vi "zad71.vi"() -> ()   [LabVIEW 2018]
uses:
  ProductsCluster.ctl
  ProductsDataToWork.ctl
  ProgramStates.ctl
  <vilib>/Utility/file.llb/Read Delimited Spreadsheet (string).vi
panel:
  in  "?":bool
  in  "SortBy":enum16{"Name", "Number", "Producer"}(ring)
  in  "?":bool
  in  "?":bool
  in  "?":bool
  in  "?":bool
  in  "Search Value":string
  in  "SearchBy":enum16{"Name", "Number", "Producer"}(ring)=enum."Number"
  in  "?":bool
  in  "?":bool
  in  "?":bool
  in  "?":bool
  out "?":T1={"Numer Produktu"="1112", "Nazwa Produktu"="Laptop", "Wytwórca"="Dell"}
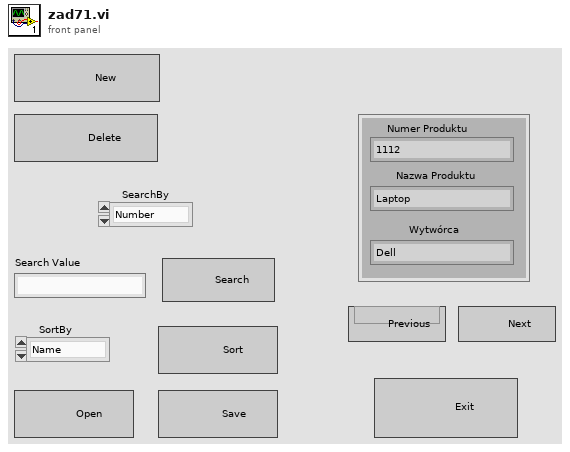
[diagram p1: front panel]
types:
  T1 = typedef "ProductsCluster.ctl" = cluster{"Numer Produktu":string, "Nazwa Produktu":string, "Wytwórca":string}
  T2 = typedef "ProductsDataToWork.ctl" = cluster{"Products":T1[], "CurrentProduct":i32, "SearchBy":enum16{"Name", "Number", "Producer"}, "SearchValue":string, "DataFilePath":path, "SortBy":enum16{"Name", "Number", "Producer"}}
  T3 = typedef "ProgramStates.ctl" = enum16{"Init", "Idle", "Open", "ShowPrevorious", "ShowNext", "Search", "Sort", "Add", "Delete", "Save", "Exit"}
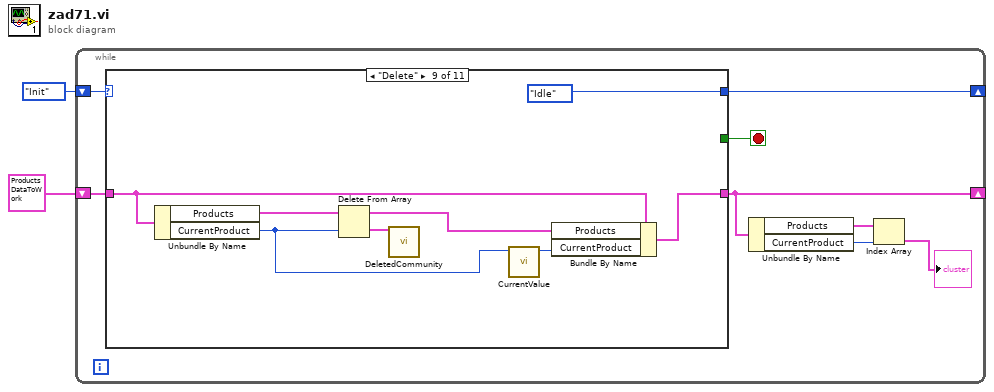
[diagram p0: block diagram]
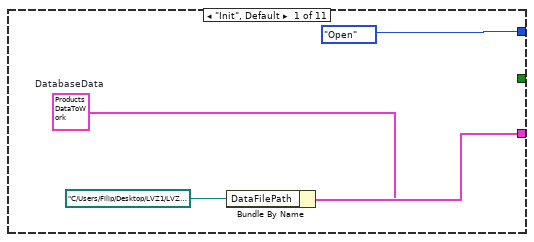
[diagram p2: hidden frame]
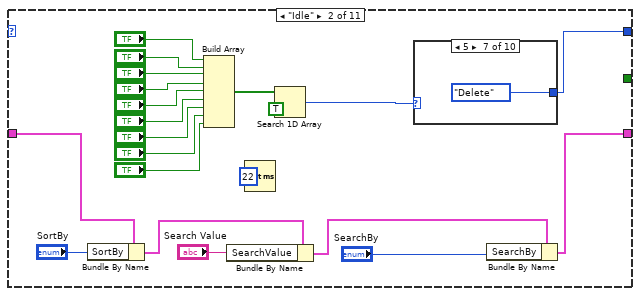
[diagram p3: hidden frame]
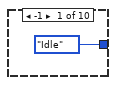
[diagram p4: hidden frame]
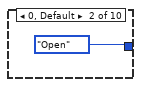
[diagram p5: hidden frame]
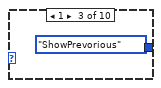
[diagram p6: hidden frame]
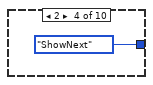
[diagram p7: hidden frame]
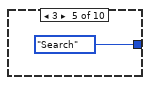
[diagram p8: hidden frame]
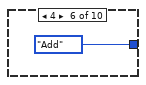
[diagram p9: hidden frame]
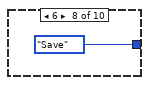
[diagram p10: hidden frame]
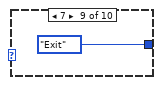
[diagram p11: hidden frame]
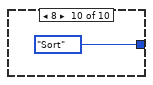
[diagram p12: hidden frame]
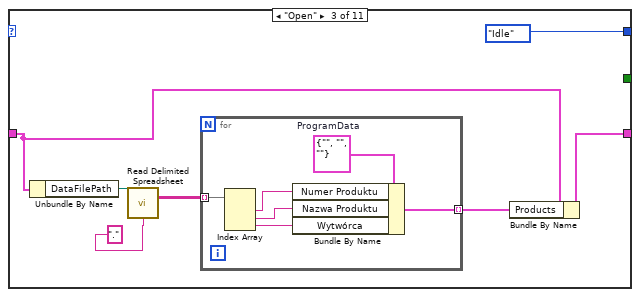
[diagram p13: hidden frame]
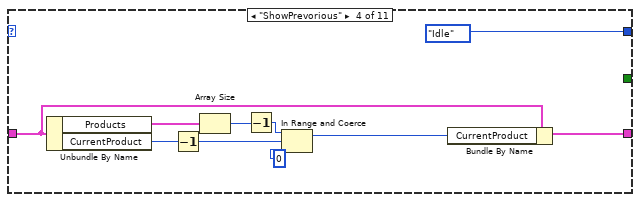
[diagram p14: hidden frame]
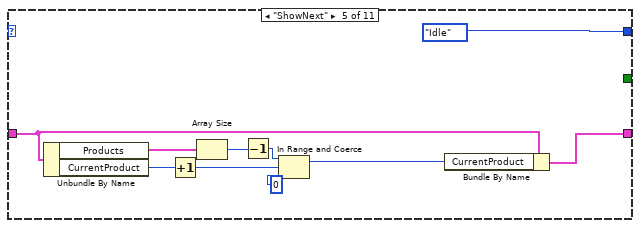
[diagram p15: hidden frame]
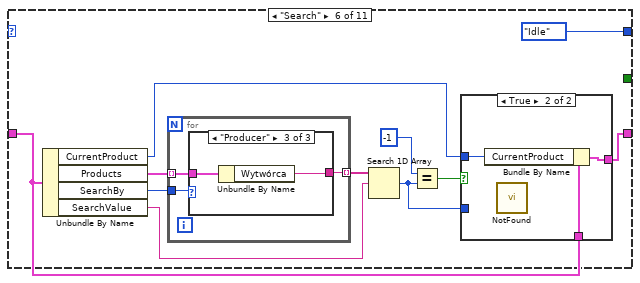
[diagram p16: hidden frame]
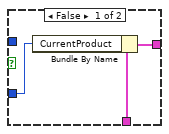
[diagram p17: hidden frame]
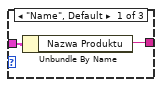
[diagram p18: hidden frame]
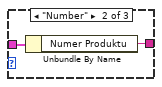
[diagram p19: hidden frame]
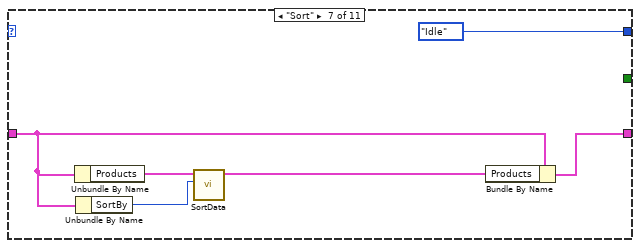
[diagram p20: hidden frame]
diagram:
  n1 = while {
    shift-right: [w5] -> _
    shift-left: T2 {"Products"=[], "CurrentProduct"=0, "SearchBy"=enum."Name", "SearchValue"="", "DataFilePath"=path "", "SortBy"=enum."Name"} ("DatabaseData") -> [w4]
    shift-right: [w7] -> _
    shift-left: ProgramStates."Init" -> [w6]
    stop <- w3 stop-if-true
    n2 = case shown="\"Delete\"" w6 {
      tunnel: [ProgramStates."Open" w21 ProgramStates."Idle" ProgramStates."Idle" ProgramStates."Idle" ProgramStates."Idle" ProgramStates."Idle" ProgramStates."Save" ProgramStates."Idle" ProgramStates."Idle" ProgramStates."Exit"] -> w7
      tunnel: [w14 w23 w52 w60 w70 w81 w110 w113 w122 w130 T2 {"Products"=[], "CurrentProduct"=0, "SearchBy"=enum."Name", "SearchValue"="", "DataFilePath"=path "", "SortBy"=enum."Name"} ("DatabaseData")] -> w5
      tunnel: w4 -> [_ w17 w46 w61 w71 w83 w107 w114 w123 w130 w134]
      tunnel: [_ _ _ _ _ _ _ _ _ _ TRUE] -> w3
      frame "Init", Default {
        w11 = T2 {"Products"=[], "CurrentProduct"=0, "SearchBy"=enum."Name", "SearchValue"="", "DataFilePath"=path "", "SortBy"=enum."Name"}  # DatabaseData
        n3 = Bundle By Name(cluster=w11, "DataFilePath"=path "C:/Users/Filip/Desktop/LVZ1/LVZ7/data.csv" ("DatabaseFilePath")) -> (w14:T2)
      }
      frame "Idle" {
        n4 = Bundle By Name(cluster=w17, "SortBy"="SortBy") -> (w16:T2)
        n5 = Build Array("?", "?", "?", "?", "?", "?", "?", "?", "?") -> (w27:bool[])
        n6 = Bundle By Name(cluster=w16, "SearchValue"="Search Value") -> (w18:T2)
        n7 = Wait (ms)(milliseconds to wait=u32 22) -> ()  [unwired: 1 out]
        n8 = Search 1D Array(1D array=w27, element=TRUE) -> (index of element=w26:i32)  [unwired: 1 in]
        n9 = case shown="5" w26 {
          tunnel: [ProgramStates."Idle" ProgramStates."Open" ProgramStates."ShowPrevorious" ProgramStates."ShowNext" ProgramStates."Search" ProgramStates."Add" ProgramStates."Delete" ProgramStates."Save" ProgramStates."Exit" ProgramStates."Sort"] -> w21
          frame -1 {
          }
          frame 0, Default {
          }
          frame 1 {
          }
          frame 2 {
          }
          frame 3 {
          }
          frame 4 {
          }
          frame 5 {
          }
          frame 6 {
          }
          frame 7 {
          }
          frame 8 {
          }
        }
        n10 = Bundle By Name(cluster=w18, "SearchBy"="SearchBy") -> (w23:T2)
      }
      frame "Open" {
        n11 = Unbundle By Name(w46) -> ("DataFilePath"=w50:path)
        n12 = call-poly <vilib>:"Read Delimited Spreadsheet.vi"("file path (dialog if empty)"=w50, "delimiter (\\t)"=".") -> ("all rows"=w48:string[][])  [unwired: 8 in, 5 out]
        n13 = for {
          tunnel: w48 -> [w58] mode=indexing
          tunnel: [w54] -> w47 mode=indexing
          w53 = T1 {"Numer Produktu"="", "Nazwa Produktu"="", "Wytwórca"=""}  # ProgramData
          n14 = Index Array(array=w58) -> (element #1=w57:string, element #2=w56:string, element #3=w55:string)  [unwired: 3 in]
          n15 = Bundle By Name(cluster=w53, "Numer Produktu"=w57, "Nazwa Produktu"=w56, "Wytwórca"=w55) -> (w54:T1)
        }
        n16 = Bundle By Name(cluster=w46, "Products"=w47) -> (w52:T2)
      }
      frame "ShowPrevorious" {
        n17 = Unbundle By Name(w61) -> ("Products"=w64:T1[], "CurrentProduct"=w63:i32)
        n18 = Decrement(x=w63) -> (x-1=w65:i32)
        n19 = Array Size(array=w64) -> (size(s)=w66:i32)
        n20 = Decrement(x=w66) -> (x-1=w67:i32)
        n21 = In Range and Coerce(upper limit=w67, x=w65, lower limit=0) -> (coerced(x)=w68:i32)  [unwired: 1 out]
        n22 = Bundle By Name(cluster=w61, "CurrentProduct"=w68) -> (w60:T2)
      }
      frame "ShowNext" {
        n23 = Unbundle By Name(w71) -> ("Products"=w74:T1[], "CurrentProduct"=w73:i32)
        n24 = Increment(x=w73) -> (x+1=w75:i32)
        n25 = Array Size(array=w74) -> (size(s)=w76:i32)
        n26 = Decrement(x=w76) -> (x-1=w77:i32)
        n27 = In Range and Coerce(upper limit=w77, x=w75, lower limit=0) -> (coerced(x)=w78:i32)  [unwired: 1 out]
        n28 = Bundle By Name(cluster=w71, "CurrentProduct"=w78) -> (w70:T2)
      }
      frame "Search" {
        n29 = Unbundle By Name(w83) -> ("CurrentProduct"=w82:i32, "Products"=w89:T1[], "SearchBy"=w87:enum16{"Name", "Number", "Producer"}, "SearchValue"=w86:string)
        n30 = for {
          tunnel: w89 -> [w98] mode=indexing
          tunnel: [w97] -> w88 mode=indexing
          tunnel: w87 -> [w96]
          n31 = case shown="\"Producer\"" w96 {
            tunnel: w98 -> [w99 w102 w104]
            tunnel: [w100 w101 w103] -> w97
            frame "Name", Default {
              n32 = Unbundle By Name(w99) -> ("Nazwa Produktu"=w100:string)
            }
            frame "Number" {
              n33 = Unbundle By Name(w102) -> ("Numer Produktu"=w101:string)
            }
            frame "Producer" {
              n34 = Unbundle By Name(w104) -> ("Wytwórca"=w103:string)
            }
          }
        }
        n35 = Search 1D Array(1D array=w88, element=w86) -> (index of element=w79:i32)  [unwired: 1 in]
        n36 = Equal?(x=-1 ("y"), y=w79) -> (x = y?=w85:bool)
        n37 = case shown="True" w85 {
          tunnel: w83 -> [w92 w95]
          tunnel: w82 -> [_ w94]
          tunnel: [w90 w93] -> w81
          tunnel: w79 -> [w91 _]
          frame False {
            n38 = Bundle By Name(cluster=w92, "CurrentProduct"=w91) -> (w90:T2)
          }
          frame True {
            n39 = Bundle By Name(cluster=w95, "CurrentProduct"=w94) -> (w93:T2)
            n40 = call "NotFound.vi"() -> ()  [unwired: 12 in]
          }
        }
      }
      frame "Sort" {
        n41 = Unbundle By Name(w107) -> ("Products"=w109:T1[])
        n42 = Unbundle By Name(w107) -> ("SortBy"=w106:enum16{"Name", "Number", "Producer"})
        n43 = call "SortData.vi"("SortBy"=w106, "ProductsToSort"=w109) -> ("ProductsSorted"=w108:T1[])  [unwired: 9 in]
        n44 = Bundle By Name(cluster=w107, "Products"=w108) -> (w110:T2)
      }
      frame "Add" {
        n45 = call "AddData.vi"() -> (2:w111:bool, "ProgramData 2"=w112:T1)  [unwired: 10 in]
        n46 = Unbundle By Name(w114) -> ("Products"=w115:T1[])
        n47 = Build Array (concatenate)(w115, w112) -> (w116:T1[])
        n48 = Select(t=w115, s=w111, f=w116) -> (s? t:f=w117:T1[])
        n49 = Bundle By Name(cluster=w114, "Products"=w117) -> (w113:T2)
      }
      frame "Delete" {
        n50 = Unbundle By Name(w123) -> ("Products"=w125:T1[], "CurrentProduct"=w119:i32)
        n51 = Delete From Array(array=w125, index=w119) -> (deleted portion=w121:T1, array with subset deleted=w124:T1[])  [unwired: 1 in]
        n52 = call "DeletedCommunity.vi"("ProgramData"=w121) -> ()  [unwired: 11 in]
        n53 = call "CurrentValue.vi"("CurrentIn"=w119) -> ("CurrentOut"=w120:i32)  [unwired: 10 in]
        n54 = Bundle By Name(cluster=w123, "Products"=w124, "CurrentProduct"=w120) -> (w122:T2)
      }
      frame "Save" {
        n55 = Unbundle By Name(w130) -> ("Products"=w128:T1[], "DataFilePath"=w127:path)
        n56 = call "SaveData.vi"("DataFilePath"=w127, "Products"=w128) -> ()  [unwired: 10 in]
      }
      frame "Exit" {
        n57 = Unbundle By Name(w134) -> ("Products"=w133:T1[], "DataFilePath"=w132:path)
        n58 = call "SaveData.vi"("DataFilePath"=w132, "Products"=w133) -> ()  [unwired: 10 in]
      }
    }
    n59 = Unbundle By Name(w5) -> ("Products"=w9:T1[], "CurrentProduct"=w10:i32)
    n60 = Index Array(array=w9, index=w10) -> (element=→"?":T1)
  }
